vi "H5Sselect_elements.vi"(6 "error in (no error)":errorcluster, 7 "Pointlist":u64[][](array[numeric]), 8 "Operator":T1 items=["H5S_SELECT_NOOP"=-1, "H5S_SELECT_SET"=0, "H5S_SELECT_OR"=1, "H5S_SELECT_AND"=2, "H5S_SELECT_XOR"=3, "H5S_SELECT_NOTB"=4, "H5S_SELECT_NOTA"=5, "H5S_SELECT_APPEND"=6, "H5S_SELECT_PREPEND"=7], 9 "HDF5 Space Ref":T2) -> (0 "error out":errorcluster, 3 "HDF5 Ref out":T2)   [LabVIEW 2017]
doc: "Selects array elements to be included in the selection for a dataspace."
uses:
  <vilib>/UPVI/lvhdf5/library.llb/HDF5 Ref.ctl
  <vilib>/UPVI/lvhdf5/dataspace.llb/H5S_seloper_t.ctl
  <vilib>/UPVI/lvhdf5/hdf5.dll
panel:
  # "LVHDF5 Toolkit\nCopyright (c) 2005-2013 by Jason D. Sommerville\nCopyright (c) 2014 by UPVI, LLC.\n\nThis use and distribution of this file is governed by the terms found in \nLICENSE.txt distributed with this toolkit and installed at\n <user.lib>\\_lvhdf5\\LICENSE.txt"
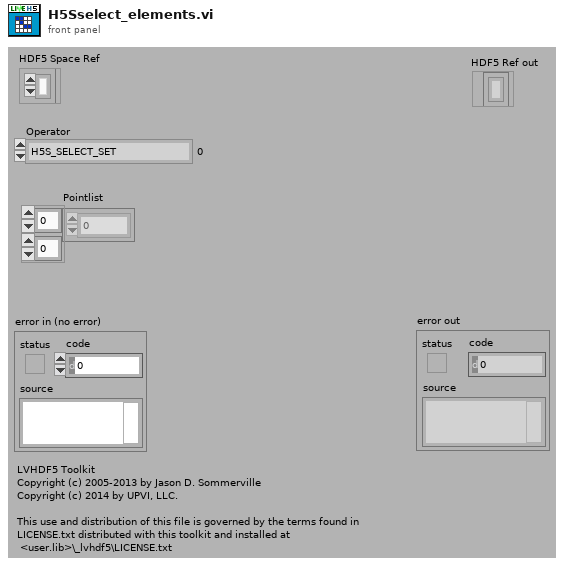
[diagram p1: front panel]
types:
  T1 = typedef "H5S_seloper_t.ctl" = i32
  T2 = typedef "HDF5 Ref.ctl" = refnum<k1>
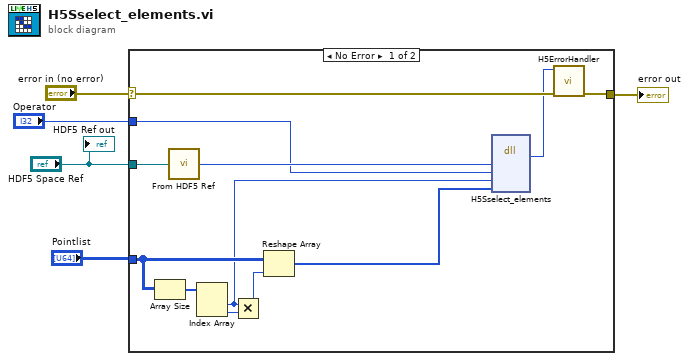
[diagram p0: block diagram]
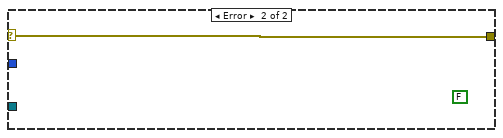
[diagram p2: hidden frame]
diagram:
  n1 = case shown="No Error" "error in (no error)" {
    selector: "error in (no error)" -> [w17 w18]
    tunnel: [w16 w18] -> w4
    tunnel: "HDF5 Space Ref" -> [w15 _]
    tunnel: "Operator" -> [w12 _]
    tunnel: "Pointlist" -> [w9 _]
    frame No Error {
      n2 = Array Size(array=w9) -> (size(s)=w10:i32[])
      n3 = call <vilib>:"From HDF5 Ref.vi"("HDF5 Ref"=w15) -> ("I32"=w14:i32)
      n4 = Index Array(array=w10) -> (element #1=w7:i32, element #2=w8:i32)  [unwired: 2 in]
      n5 = Multiply(x=w7, y=w8) -> (x*y=w11:i32)
      n6 = Reshape Array(w9, w11) -> (w6:u64[])
      n7 = dll-call lib="C:/Program Files/National Instruments/LabVIEW 2017/vi.lib/UPVI/lvhdf5/hdf5.dll" fn="H5Sselect_elements"("space_id"=w14, "op"=w12, "num_elements"=w7, "coord"=w6) -> ("return type"=w13:i32)  [unwired: 7 in, 2 out]
      n8 = call <vilib>:"H5ErrorHandler.vi"("error in (no error)"=w17, "herr_t"=w13) -> ("error out"=w16:errorcluster)  [unwired: 3 in, 4 out]
    }
    frame Error {
      (unwired) FALSE
    }
  }
  "error out" <- w4
  "HDF5 Ref out" <- "HDF5 Space Ref"
